vi "RGB_tot.vi"(2 "error in":errorcluster, 3 "output array":u16[][](array[numeric]), 4 "SCI":u8) -> (0 "error out":errorcluster)   [LabVIEW 2013]
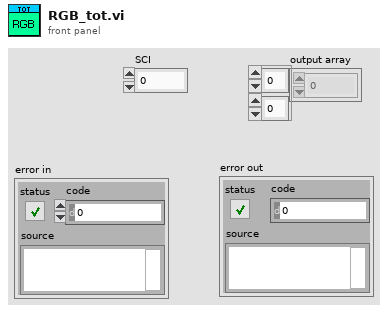
[diagram p1: front panel]
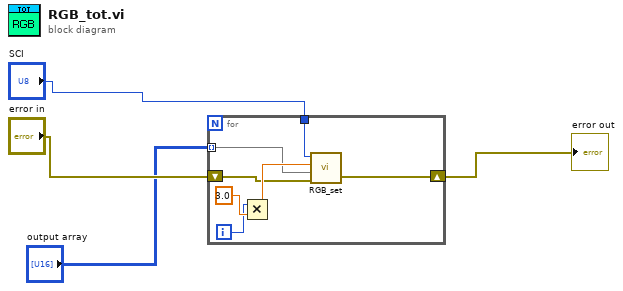
[diagram p0: block diagram]
diagram:
  n1 = for {
    shift-right: [w8] -> w3
    shift-left: "error in" -> [w6]
    tunnel: "output array" -> [w5] mode=indexing
    tunnel: "SCI" -> [w7]
    i -> [w10]
    n2 = Multiply(x=w10, y=3.0) -> (x*y=w9:dbl)
    n3 = call "RGB_set.vi"("error in"=w6, "RGB"=w5, "Channel_start"=w9, "SCI"=w7) -> ("error out"=w8:errorcluster)  [unwired: 1 in]
  }
  "error out" <- w3
